vi "Send State Change Core.vi"(7 "Message Priority (Normal)":T1=enum."Normal", 8 "error in (no error)":errorcluster, 10 "Transition State":refnum<class "State Change Core.lvclass">, 11 "Message Enqueuer":refnum<class "Message Enqueuer.lvclass">) -> (0 "error out":errorcluster, 3 "Message Enqueuer out":refnum<class "Message Enqueuer.lvclass">)   [LabVIEW 2021, in "State Change Core.lvlib" / "State Change Core Msg.lvclass"]
doc: "This VI sends the message to an actor."
uses:
  State Change Core Msg.lvclass
  State Change Core Msg.lvclass/State Change Core Msg.ctl
  <vilib>/ActorFramework/Message Enqueuer/Message Enqueuer.lvclass
  C:/Program Files/National Instruments/LabVIEW 2021/vi.lib/ActorFramework/Message/Message.lvclass
  C:/PPLs/Design-Patterns/State Pattern/State Change Core/State Change Core Messages/State Change Core Msg/State Change Core Msg.lvclass
  <vilib>/ActorFramework/Message Enqueuer/Message Priority.ctl
  State Change Core/State Change Core.lvclass
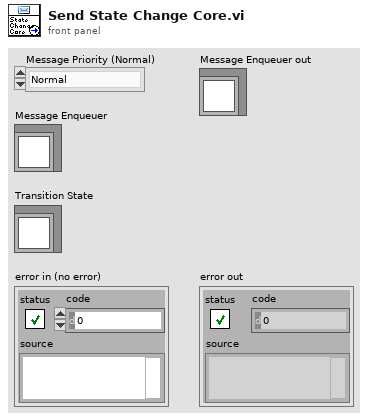
[diagram p1: front panel]
types:
  T1 = typedef "Actor Framework.lvlib/Message Enqueuer.lvclass/Message Priority.ctl" = enum16{"Low", "Normal", "High"}
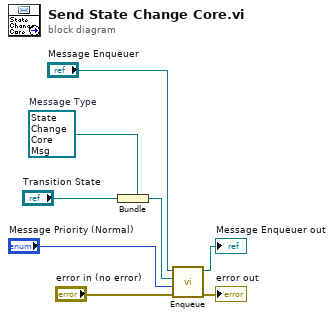
[diagram p0: block diagram]
diagram:
  w5 = refnum<class "State Change Core Msg.lvclass"> refnum  # Message Type
  n1 = Bundle(cluster=w5, "Transition State") -> (w4:refnum<class "State Change Core Msg.lvclass">)
  n2 = call <vilib>:"Enqueue.vi"("error in (no error)"="error in (no error)", "Message Priority (Normal)"="Message Priority (Normal)", "Message"=w4, "Message Enqueuer in"="Message Enqueuer") -> ("error out"=→"error out":errorcluster, "Message Enqueuer in"=→"Message Enqueuer out":refnum<class "Message Enqueuer.lvclass">)  [unwired: 6 in]
